vi "PID_TempControl_GCFS.vi"(8 "error in":errorcluster, 9 "CheckResponse?":bool, 10 "Manual Temp Control.Active":bool, 11 "?":T2 {"Data Out Cluster"."Particle Measurements (Pixels) (Particle Analysis 1)" format="%.2f"}) -> (0 "error out":errorcluster, 1 "date/time string":string, 2 "Image Out":T1, 3 "Temperature":dbl, 4 "Output%":dbl format="%.2f", 5 "valid?":bool, 6 "Temp Gradient":dbl)   [LabVIEW 2024]
uses:
  DataCluster_GCFS.ctl
  <vilib>/userDefined/High Color/IMAQdx.ctl
  <vilib>/vision/Image Controls.llb/IMAQ Image.ctl
  ee7b73c5-abbe-409c-97f6-86d988c3f229.vi
  <vilib>/addons/control/pid/pid.llb/PID (DBL).vi
  <vilib>/regexp/Match Regular Expression.xnode
  <vilib>/addons/control/pid/NI_PID_pid.lvlib
panel:
  in  "Data Acquisition.Setup.TempGrad":dbl
  in  "reinitialize? (F)":bool
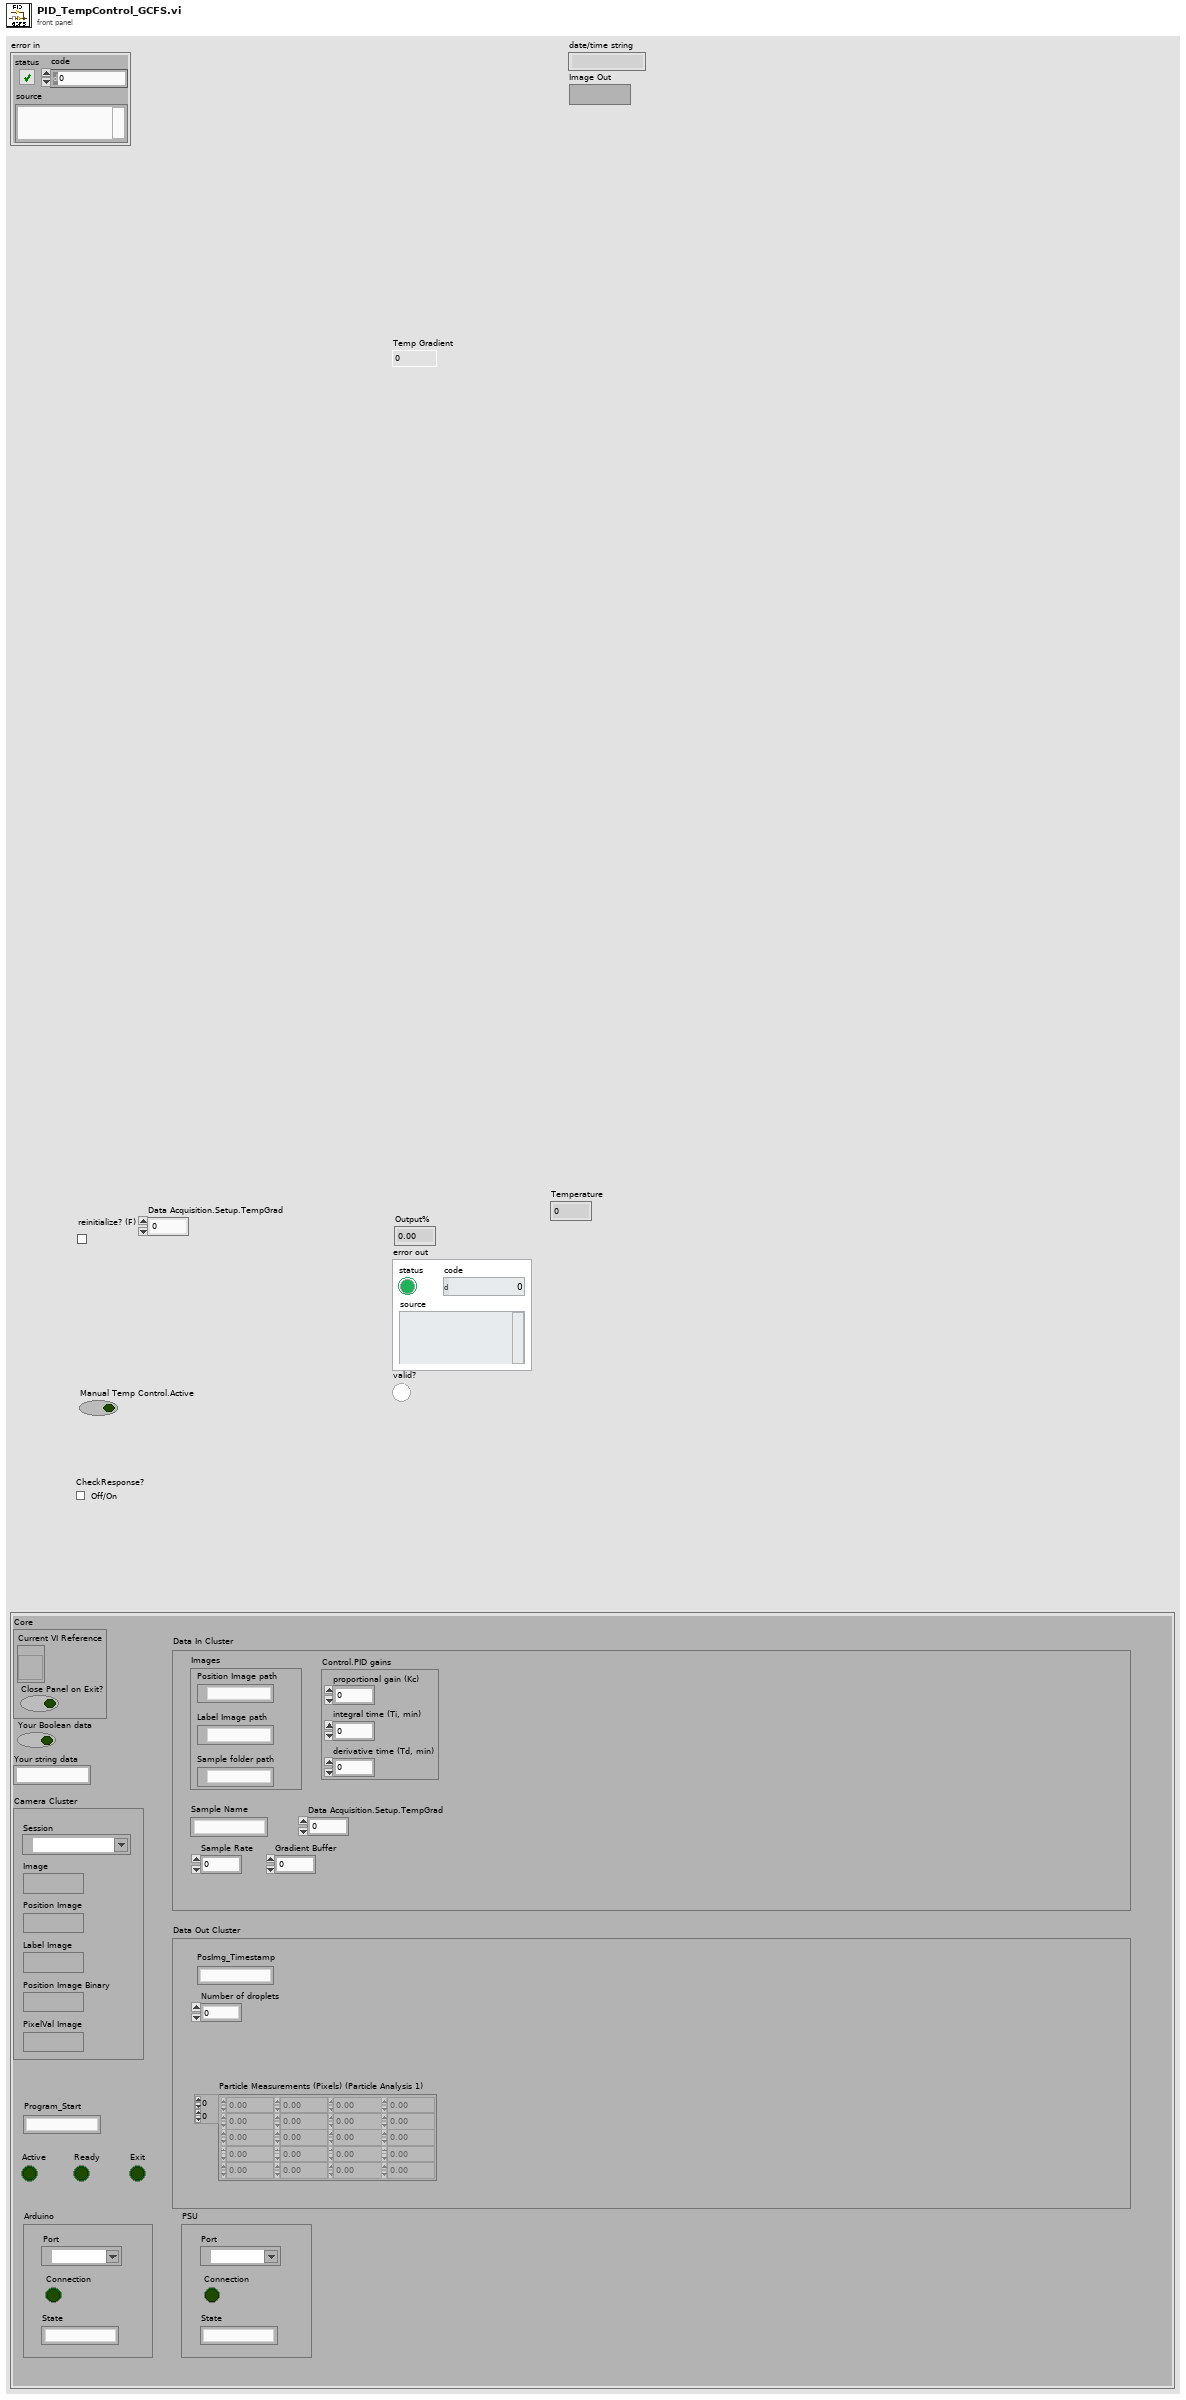
[diagram p1: front panel]
types:
  T1 = typedef "IMAQ Image.ctl" = refnum<image>
  T2 = typedef "DataCluster_GCFS.ctl" = cluster{"Core":cluster{"Current VI Reference":refnum<vi>, "Close Panel on Exit?":bool}, "Your Boolean data":bool, "Your string data":string, "Camera Cluster":cluster{"Session":T3, "Image":T1, "Position Image":T1, "PixelVal Image":T1, "Position Image Binary":T1, "Lable Image":T1}, "Data In Cluster":cluster{"Images":cluster{"Position Image path":path, "Sample folder path":path, "Label Image path":path}, "Sample Name":string, "Sample Rate":i32, "Gradient Buffer":i32, "Data Acquisition.Setup.TempGrad":dbl, "Control.PID gains":cluster{"proportional gain (Kc)":dbl, "integral time (Ti, min)":dbl, "derivative time (Td, min)":dbl}}, "Active":bool, "Ready":bool, "Exit":bool, "Arduino":cluster{"Connection":bool, "Port":refnum<visa-resource-name>, "State":string}, "Program_Start":string, "Data Out Cluster":cluster{"Particle Measurements (Pixels) (Particle Analysis 1)":dbl[][], "Number of droplets":i32, "PosImg_Timestamp":string}, "PSU":cluster{"Connection":bool, "Port":refnum<visa-resource-name>, "State":string}}
  T3 = typedef "IMAQdx.ctl" = refnum<k21>
  T4 = cluster{"proportional gain (Kc)":dbl, "integral time (Ti, min)":dbl, "derivative time (Td, min)":dbl}
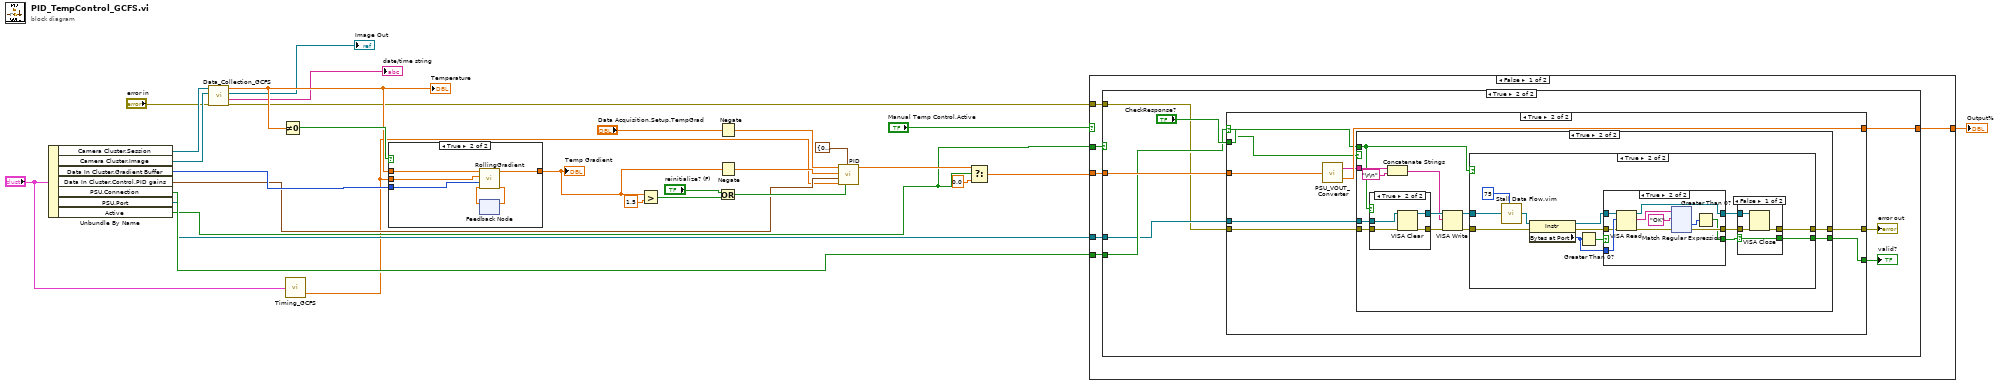
[diagram p0: block diagram]
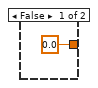
[diagram p2: hidden frame]
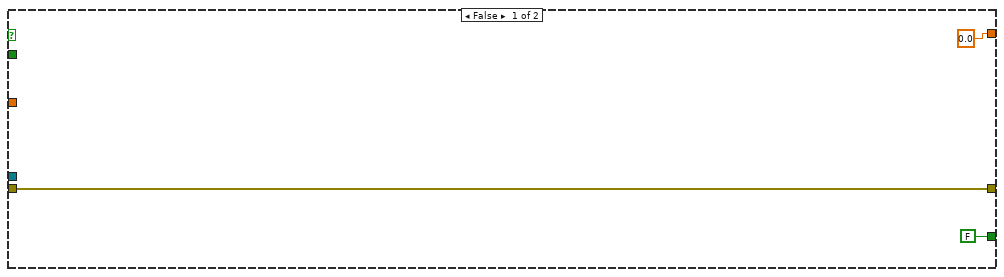
[diagram p3: hidden frame]
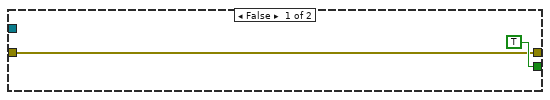
[diagram p6: hidden frame]
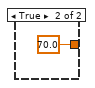
[diagram p9: hidden frame]
diagram:
  n1 = Unbundle By Name("?") -> ("Camera Cluster.Session"=w13:T3, "Camera Cluster.Image"=w12:T1, "Data In Cluster.Gradient Buffer"=w11:i32, "Data In Cluster.Control.PID gains"=w10:T4, "PSU.Connection"=w9:bool, "PSU.Port"=w8:refnum<visa-resource-name>, "Active"=w3:bool)
  n2 = call "Data_Collection_GCFS.vi"("error in"="error in", "Image"=w12, "Session"=w13) -> ("error out"=w7:errorcluster, "date/time string"=→"date/time string":string, "Image Out"=→"Image Out":T1, "Temperature"=w28:dbl)  [unwired: 5 in]
  "Temperature" <- w28
  n3 = Not Equal To 0?(x=w28) -> (x != 0?=w29:bool)
  n4 = call "Timing_GCFS.vi"(0:"?") -> ("Sample dt (s)"=w1:dbl)  [unwired: 1 out]
  n5 = case shown="True" w29 {
    tunnel: w1 -> [_ w34]
    tunnel: [_ w33] -> w18
    tunnel: w28 -> [_ w35]
    tunnel: w11 -> [_ w32]
    frame False {
    }
    frame True {
      n6 = feedback #1() -> (w31:dbl[])  [unwired: 1 in]
      n7 = call "RollingGradient.vi"("TempArray in"=w31, "FitSize"=w32, "dt"=w34, "mean temp"=w35) -> ("TempArray"=w30:dbl[], "gradient"=w33:dbl)  [unwired: 6 in]
      n8 = feedback-in #1(w30) -> ()
    }
  }
  "Temp Gradient" <- w18
  n9 = Greater?(x=w18, y=1.5) -> (0:w26:bool)
  n10 = Negate(x="Data Acquisition.Setup.TempGrad") -> (-x=w23:dbl)
  n11 = Negate(x=w18) -> (-x=w20:dbl)
  n12 = Or(x="reinitialize? (F)", y=w26) -> (x .or. y?=w17:bool)
  n13 = call-poly <vilib>:"PID.vi"("reinitialize? (F)"=w17, "output range"=cluster{"output high":dbl, "output low":dbl} {"output high"=0.0, "output low"=100.0}, "dt (s)"=w1, "PID gains"=w10, "process variable"=w20, "setpoint"=w23) -> ("output"=w19:dbl)  [unwired: 4 in, 1 out]
  n14 = Select(t=w19, s=w3, f=0.0) -> (s? t:f=w16:dbl)
  n15 = case shown="False" "Manual Temp Control.Active" {
    tunnel: w16 -> [w41 _]
    tunnel: [w40 70.0 ("Output % duplicate")] -> w24
    tunnel: w3 -> [w39 _]
    tunnel: w9 -> [w38 _]
    tunnel: w8 -> [w37 _]
    tunnel: w7 -> [w36 _]
    frame False {
      n16 = case shown="True" w39 {
        tunnel: w41 -> [_ w47]
        tunnel: [0.0 ("Output % duplicate") w46] -> w40
        tunnel: w38 -> [_ w45]
        tunnel: w37 -> [_ w44]
        tunnel: w36 -> [_ w43]
        frame False {
        }
        frame True {
          n17 = case shown="True" w45 {
            selector: w45 -> [_ w55]
            tunnel: w47 -> [_ w62]
            tunnel: [0.0 ("Output % duplicate") w61] -> w46
            tunnel: w43 -> [w51 w58]
            tunnel: [w51 w56] -> w50
            tunnel: [FALSE ("valid?") w57] -> w49
            tunnel: "CheckResponse?" -> [_ w59]
            tunnel: w44 -> [_ w54]
            frame False {
            }
            frame True {
              n18 = call "PSU_VOUT_Converter.vi"("Output %"=w62) -> ("decimal integer string"=w60:string, "Output % duplicate"=w61:dbl)
              n19 = case shown="True" w55 {
                selector: w55 -> [w63 _]
                tunnel: w54 -> [_ w75]
                tunnel: w58 -> [w64 w74]
                tunnel: [w64 w68] -> w56
                tunnel: [w63 w67] -> w57
                tunnel: w60 -> [_ w69]
                tunnel: w59 -> [_ w66]
                frame False {
                }
                frame True {
                  n20 = case shown="True" w66 {
                    tunnel: w75 -> [w78 w82]
                    tunnel: w74 -> [w77 w81]
                    tunnel: [w78 w80] -> w73
                    tunnel: [w77 w79] -> w72
                    frame False {
                    }
                    frame True {
                      n21 = VISA Clear(VISA resource name=w82, error in (no error)=w81) -> (VISA resource name out=w80:refnum<visa-resource-name>, error out=w79:errorcluster)
                    }
                  }
                  n22 = Concatenate Strings(w69, "\r\n") -> (w65:string)
                  n23 = VISA Write(VISA resource name=w73, write buffer=w65, error in (no error)=w72) -> (VISA resource name out=w71:refnum<visa-resource-name>, error out=w70:errorcluster)  [unwired: 1 out]
                  n24 = case shown="True" w66 {
                    tunnel: w71 -> [_ w91]
                    tunnel: w70 -> [w83 w90]
                    tunnel: [w83 w88] -> w68
                    tunnel: [TRUE w86] -> w67
                    frame False {
                    }
                    frame True {
                      n25 = call "Stall Data Flow.vim"("value in"=w91, "milliseconds to wait"=u32 75) -> ("value out"=w97:refnum<visa-resource-name>)  [unwired: 1 out]
                      n26 = property class="Instr"(reference=w97, error in=w90) -> (reference out=w94:refnum<visa-resource-name>, error out=w93:errorcluster, "Bytes at Port"=w95:u32)
                      n27 = Greater Than 0?(x=w95) -> (x > 0?=w96:bool)
                      n28 = case shown="True" w96 {
                        selector: w96 -> [w105 _]
                        tunnel: w95 -> [_ w116]
                        tunnel: w93 -> [w106 w115]
                        tunnel: [w106 w110] -> w87
                        tunnel: w94 -> [w104 w114]
                        tunnel: [w105 w108] -> w89
                        tunnel: [w104 w107] -> w85
                        frame False {
                        }
                        frame True {
                          n29 = VISA Read(VISA resource name=w114, byte count=w116, error in (no error)=w115) -> (VISA resource name out=w107:refnum<visa-resource-name>, read buffer=w113:string, error out=w112:errorcluster)  [unwired: 1 out]
                          n30 = xnode "Match Regular Expression"("input string"=w113, "regular expression"="OK", "error in"=w112) -> ("offset past match"=w109:i32, "error out"=w110:errorcluster)  [unwired: 3 in, 3 out]
                          n31 = Greater Than 0?(x=w109) -> (x > 0?=w108:bool)
                        }
                      }
                      n32 = case shown="False" w89 {
                        selector: w89 -> [w101 w102]
                        tunnel: [w98 w103] -> w88
                        tunnel: w87 -> [w99 w103]
                        tunnel: [w101 w102] -> w86
                        tunnel: w85 -> [w100 _]
                        frame False {
                          n33 = VISA Close(VISA resource name=w100, error in (no error)=w99) -> (error out=w98:errorcluster)
                        }
                        frame True {
                        }
                      }
                    }
                  }
                }
              }
            }
          }
          "error out" <- w50
          "valid?" <- w49
        }
      }
    }
    frame True {
    }
  }
  "Output%" <- w24
